vi "Feeding_OPEN_DOOR_ON_SCAN.vi"(7 "CYCLE DATA IN":T1, 8 "error in (no error)":errorcluster, 11 "raw scan code":string) -> (0 "error out":errorcluster, 2 "search valid ?":bool, 5 "CYCLE DATA OUT":T1)   [LabVIEW 2017]
uses:
  Controls/Feed_Cyc_Data.ctl
  <vilib>/Utility/file.llb/Read Delimited Spreadsheet (string).vi
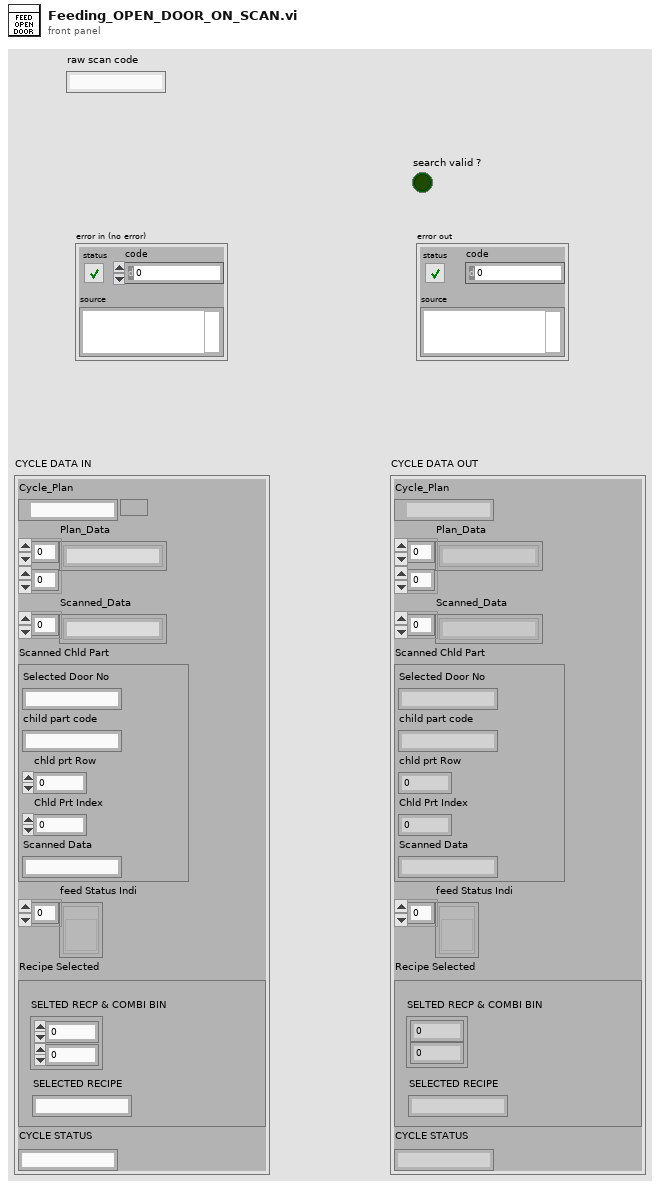
[diagram p1: front panel]
types:
  T1 = typedef "Feed_Cyc_Data.ctl" = cluster{"Cycle_Plan":path, "Plan_Data":string[][], "Scanned_Data":string[], "Scanned Chld Part":cluster{"Selected Door No":string, "child part code":string, "chld prt Row":i32, "Chld Prt Index":i32, "Scanned Data":string}, "feed Status Indi":refnum<vi>[], "Recipe Selected":cluster{"SELTED RECP & COMBI BIN":cluster{i32, i32}, "SELECTED RECIPE":string}, "CYCLE STATUS":string}
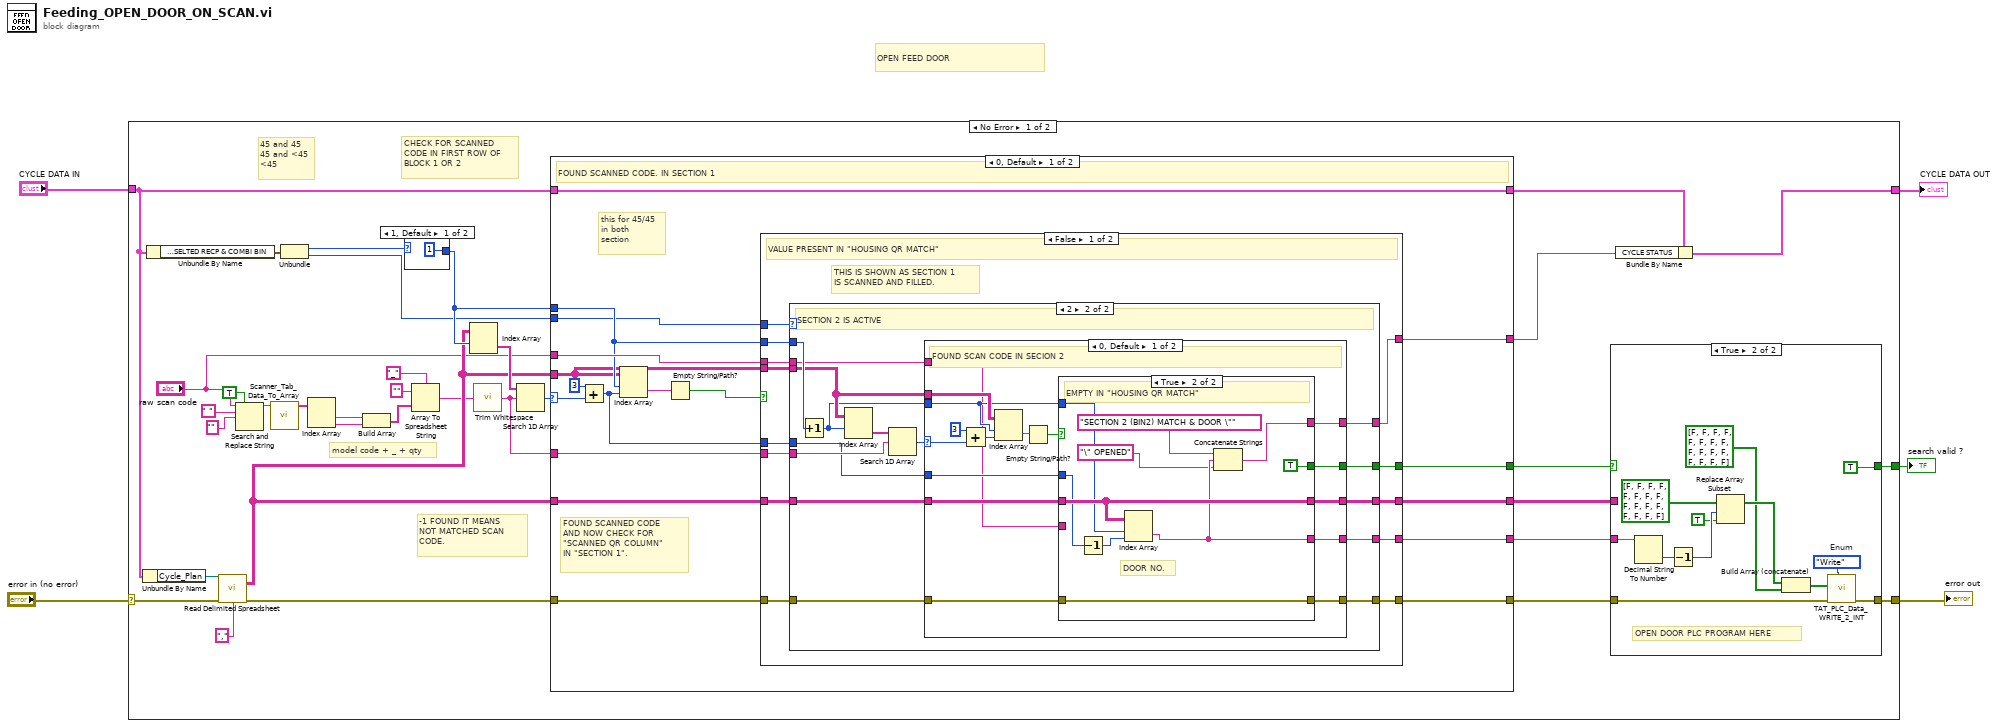
[diagram p0: block diagram]
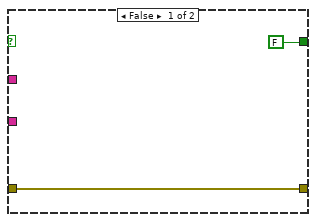
[diagram p2: hidden frame]
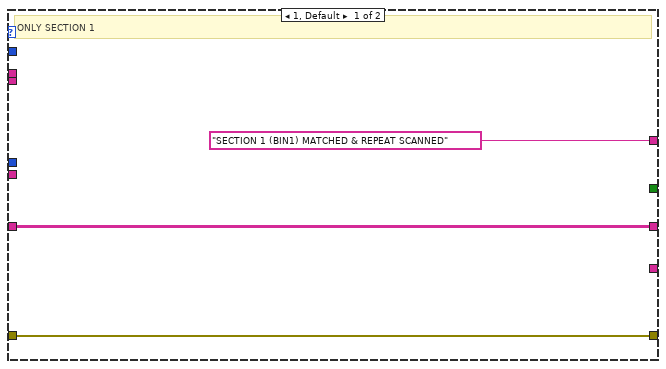
[diagram p3: hidden frame]
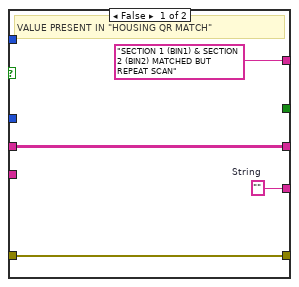
[diagram p4: hidden frame]
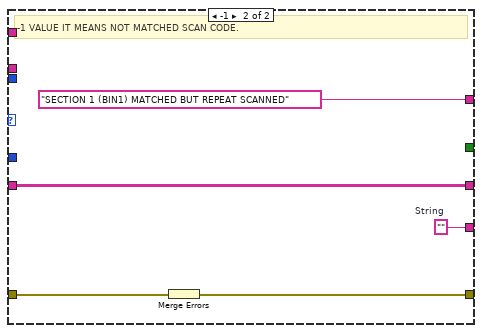
[diagram p5: hidden frame]
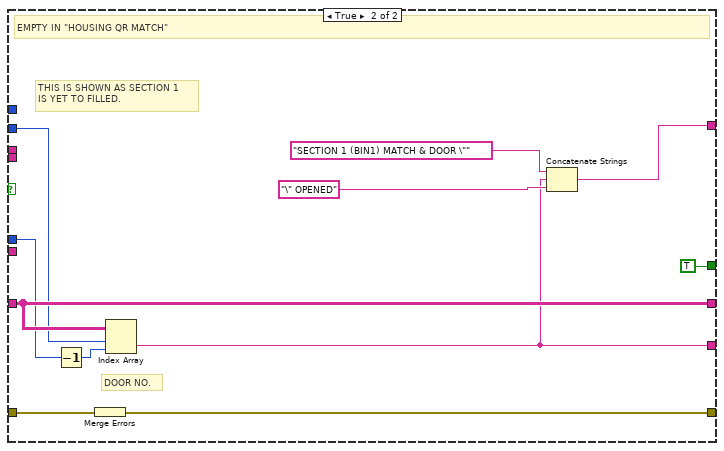
[diagram p6: hidden frame]
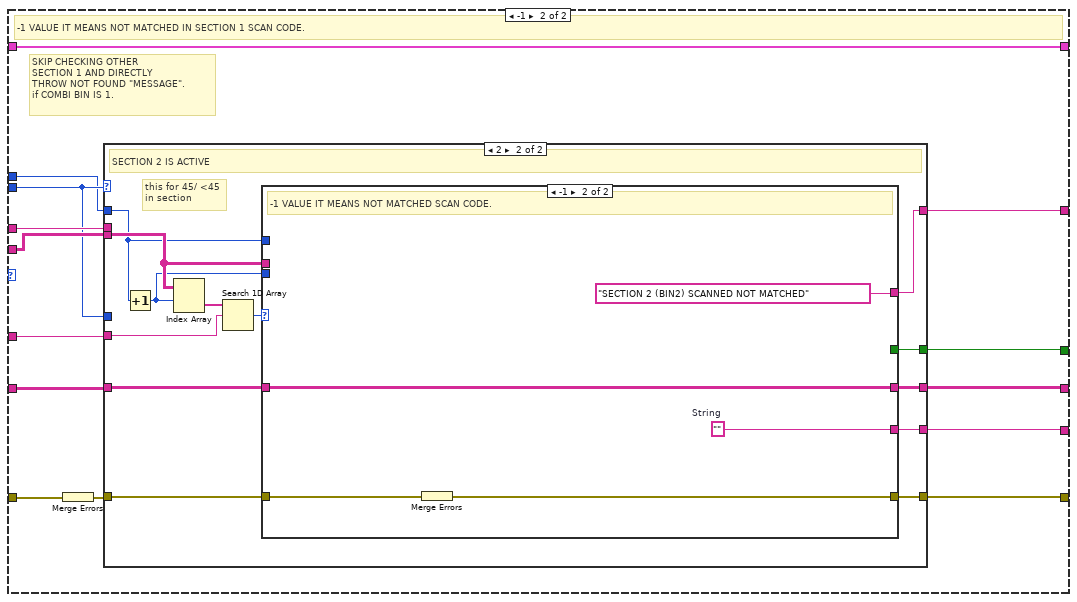
[diagram p7: hidden frame]
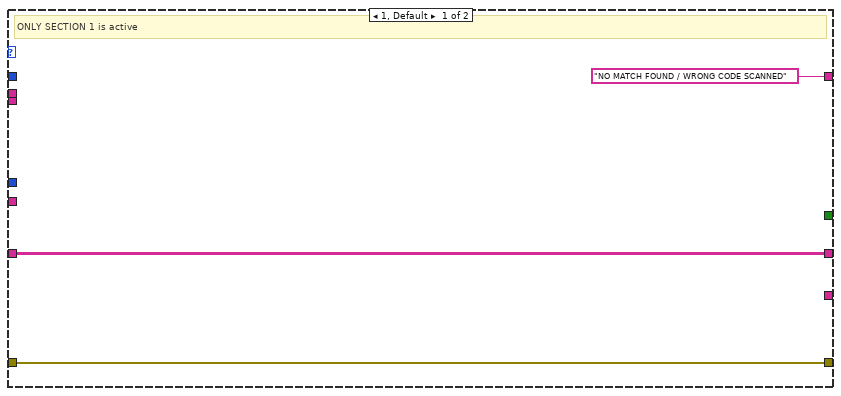
[diagram p8: hidden frame]
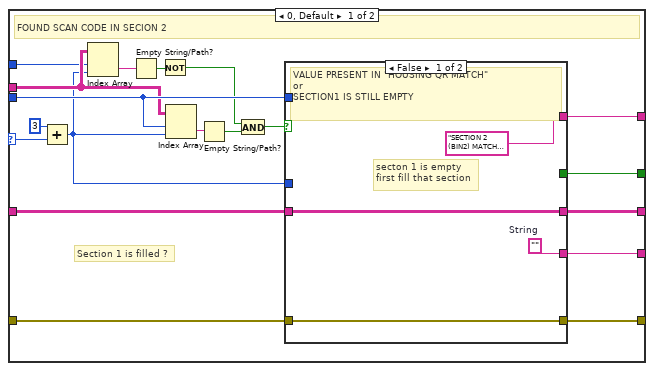
[diagram p9: hidden frame]
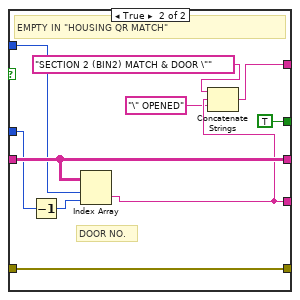
[diagram p10: hidden frame]
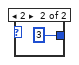
[diagram p11: hidden frame]
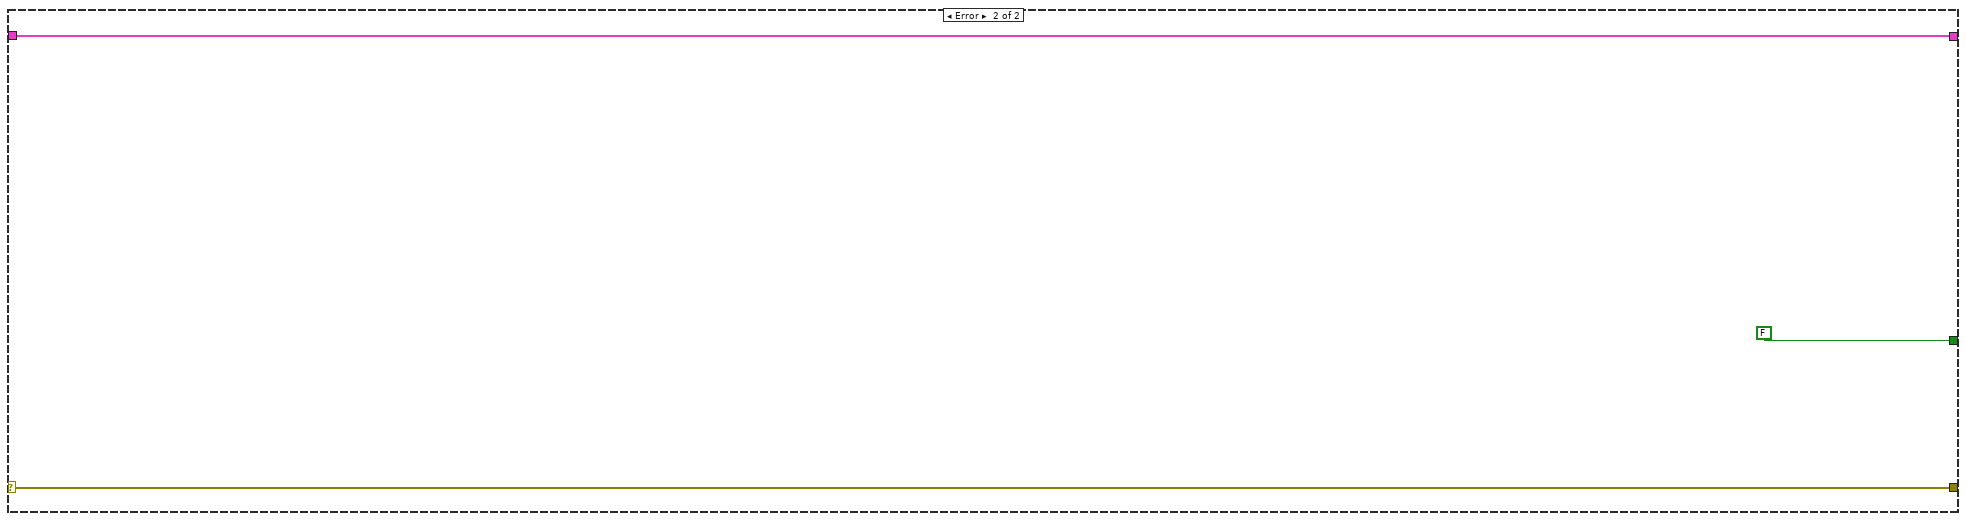
[diagram p12: hidden frame]
diagram:
  # "OPEN FEED DOOR"
  n1 = case shown="No Error" "error in (no error)" {
    selector: "error in (no error)" -> [w36 w221]
    tunnel: [w20 w221] -> w4
    tunnel: [w7 w220] -> w2
    tunnel: "CYCLE DATA IN" -> [w25 w220]
    tunnel: [w11 FALSE] -> w1
    frame No Error {
      # "45 and 45\n45 and <45\n<45"
      # "model code + _ + qty"
      # "-1 FOUND IT MEANS\nNOT MATCHED SCAN\nCODE."
      # "CHECK FOR SCANNED\nCODE IN FIRST ROW OF\nBLOCK 1 OR 2"
      n2 = Unbundle By Name(w25) -> ("Cycle_Plan"=w37:path)
      n3 = Unbundle By Name(w25) -> ("Recipe Selected.SELTED RECP & COMBI BIN"=w34:cluster{i32, i32})
      n4 = call-poly <vilib>:"Read Delimited Spreadsheet.vi"("file path (dialog if empty)"=w37, "error in (no error)"=w36, "delimiter (\\t)"=",") -> ("all rows"=w22:string[][], "error out"=w35:errorcluster)  [unwired: 7 in, 4 out]
      n5 = Search and Replace String(replace all?=TRUE, input string="raw scan code", search string=" ", replace string="") -> (result string=w32:string)  [unwired: 4 in, 3 out]
      n6 = call "Scanner_Tab_Data_To_Array.vi"("Scanner Data"=w32) -> ("Array"=w17:string[])  [unwired: 10 in]
      n7 = Unbundle(w34) -> (w33:i32, w21:i32)
      n8 = Index Array(array=w17) -> (element #1=w16:string, element #2=w15:string)  [unwired: 2 in]
      n9 = Build Array(w16, w15) -> (w14:string[])
      n10 = case shown="1, Default" w33 {
        tunnel: [1 3] -> w23
        frame 1, Default {
        }
        frame 2 {
        }
      }
      n11 = Array To Spreadsheet String(delimiter (Tab)="_", array=w14, 3:"") -> (spreadsheet string=w13:string)
      n12 = Index Array(array=w22, index (row)=w23) -> (element=w26:string[])  [unwired: 1 in]
      n13 = call <vilib>:"Trim Whitespace.vi"("string"=w13) -> ("trimmed string"=w9:string)  [unwired: 1 in]
      n14 = Search 1D Array(1D array=w26, element=w9) -> (index of element=w24:i32)  [unwired: 1 in]
      n15 = case shown="0, Default" w24 {
        selector: w24 -> [w70 _]
        tunnel: [w67 w158] -> w39
        tunnel: w35 -> [w71 w162]
        tunnel: [w64 w161] -> w8
        tunnel: w25 -> [w64 w161]
        tunnel: w22 -> [w58 w153]
        tunnel: w23 -> [w62 w150]
        tunnel: "raw scan code" -> [w65 w154]
        tunnel: w22 -> [w63 w160]
        tunnel: [w60 w156] -> w18
        tunnel: w21 -> [w59 w152]
        tunnel: w9 -> [w57 w151]
        tunnel: [w56 w155] -> w19
        tunnel: [w55 w157] -> w12
        tunnel: [w54 w149] -> w6
        frame 0, Default {
          # "this for 45/45\nin both\nsection"
          # "FOUND SCANNED CODE\nAND NOW CHECK FOR\n\"SCANNED QR COLUMN\"\nIN \"SECTION 1\"."
          # "FOUND SCANNED CODE. IN SECTION 1"
          n16 = Add(x=3, y=w70) -> (x+y=w61:i32)
          n17 = Index Array(array=w58, index (row)=w62, index (col)=w61) -> (element=w68:string)
          n18 = Empty String/Path?(string/path=w68) -> (empty?=w66:bool)
          n19 = case shown="False" w66 {
            tunnel: w71 -> [w83 w148]
            tunnel: [w84 w147] -> w67
            tunnel: w65 -> [w75 _]
            tunnel: w63 -> [w80 w146]
            tunnel: w62 -> [w79 w144]
            tunnel: w61 -> [w77 w143]
            tunnel: [w81 w146] -> w60
            tunnel: w59 -> [w82 _]
            tunnel: w58 -> [w78 _]
            tunnel: w57 -> [w76 _]
            tunnel: [w74 TRUE] -> w56
            tunnel: [w73 w139] -> w55
            tunnel: [w72 w138] -> w54
            frame False {
              # "THIS IS SHOWN AS SECTION 1\nIS SCANNED AND FILLED."
              # "VALUE PRESENT IN \"HOUSING QR MATCH\""
              n20 = case shown="2" w82 {
                tunnel: [w87 w98] -> w84
                tunnel: w83 -> [w87 w102]
                tunnel: [w86 w97] -> w81
                tunnel: w80 -> [w86 w96]
                tunnel: w79 -> [_ w101]
                tunnel: w78 -> [_ w94]
                tunnel: w77 -> [_ w92]
                tunnel: w76 -> [_ w99]
                tunnel: w75 -> [_ w91]
                tunnel: [_ w90] -> w74
                tunnel: [_ w89] -> w73
                tunnel: ["SECTION 1 (BIN1) MATCHED & REPEAT SCANNED" w88] -> w72
                frame 1, Default {
                  # "ONLY SECTION 1"
                }
                frame 2 {
                  # "SECTION 2 IS ACTIVE"
                  n21 = Increment(x=w101) -> (x+1=w93:i32)
                  n22 = Index Array(array=w94, index (row)=w93) -> (element=w100:string[])  [unwired: 1 in]
                  n23 = Search 1D Array(1D array=w100, element=w99) -> (index of element=w95:i32)  [unwired: 1 in]
                  n24 = case shown="0, Default" w95 {
                    selector: w95 -> [w115 _]
                    tunnel: w102 -> [w118 w137]
                    tunnel: [w113 w136] -> w98
                    tunnel: [w110 w135] -> w97
                    tunnel: w96 -> [w109 w135]
                    tunnel: w94 -> [w114 _]
                    tunnel: w93 -> [w108 _]
                    tunnel: w92 -> [w107 _]
                    tunnel: w91 -> [w106 _]
                    tunnel: [w105 _] -> w90
                    tunnel: [w104 w134] -> w89
                    tunnel: [w103 "SECTION 1 (BIN1) MATCHED BUT REPEAT SCANNED"] -> w88
                    frame 0, Default {
                      # "FOUND SCAN CODE IN SECION 2"
                      n25 = Add(x=3, y=w115) -> (x+y=w117:i32)
                      n26 = Index Array(array=w114, index (row)=w108, index (col)=w117) -> (element=w112:string)
                      n27 = Empty String/Path?(string/path=w112) -> (empty?=w111:bool)
                      n28 = case shown="True" w111 {
                        tunnel: w118 -> [w121 w132]
                        tunnel: [w121 w132] -> w113
                        tunnel: [w122 w129] -> w110
                        tunnel: w109 -> [w122 w129]
                        tunnel: w108 -> [_ w128]
                        tunnel: w107 -> [_ w127]
                        tunnel: w106 -> [_ _]
                        tunnel: [_ TRUE] -> w105
                        tunnel: [w120 w125] -> w104
                        tunnel: ["SECTION 1 (BIN1) & SECTION 2 (BIN2) MATCHED BUT REPEAT SCAN" w123] -> w103
                        frame False {
                          w120 = ""  # String
                          # "VALUE PRESENT IN \"HOUSING QR MATCH\""
                        }
                        frame True {
                          # "DOOR NO."
                          # "EMPTY IN \"HOUSING QR MATCH\""
                          n29 = Decrement(x=w127) -> (x-1=w130:i32)
                          n30 = Index Array(array=w129, index (row)=w128, index (col)=w130) -> (element=w125:string)
                          n31 = Concatenate Strings("SECTION 2 (BIN2) MATCH & DOOR \"", w125, "\" OPENED") -> (w123:string)
                        }
                      }
                    }
                    frame -1 {
                      w134 = ""  # String
                      # "-1 VALUE IT MEANS NOT MATCHED SCAN CODE."
                      n32 = Merge Errors(w137) -> (w136:errorcluster)
                    }
                  }
                }
              }
            }
            frame True {
              # "DOOR NO."
              # "THIS IS SHOWN AS SECTION 1\nIS YET TO FILLED."
              # "EMPTY IN \"HOUSING QR MATCH\""
              n33 = Decrement(x=w143) -> (x-1=w142:i32)
              n34 = Merge Errors(w148) -> (w147:errorcluster)
              n35 = Index Array(array=w146, index (row)=w144, index (col)=w142) -> (element=w139:string)
              n36 = Concatenate Strings("SECTION 1 (BIN1) MATCH & DOOR \"", w139, "\" OPENED") -> (w138:string)
            }
          }
        }
        frame -1 {
          # "SKIP CHECKING OTHER \nSECTION 1 AND DIRECTLY\nTHROW NOT FOUND \"MESSAGE\". \nif COMBI BIN IS 1."
          # "-1 VALUE IT MEANS NOT MATCHED IN SECTION 1 SCAN CODE."
          n37 = Merge Errors(w162) -> (w159:errorcluster)
          n38 = case shown="2" w152 {
            tunnel: [w165 w176] -> w158
            tunnel: w159 -> [w165 w178]
            tunnel: [w164 w175] -> w156
            tunnel: w160 -> [w164 w174]
            tunnel: w153 -> [_ w171]
            tunnel: w152 -> [_ _]
            tunnel: w151 -> [_ w177]
            tunnel: w154 -> [_ _]
            tunnel: [_ w173] -> w155
            tunnel: [_ w172] -> w157
            tunnel: w150 -> [_ w167]
            tunnel: ["NO MATCH FOUND / WRONG CODE SCANNED" w166] -> w149
            frame 1, Default {
              # "ONLY SECTION 1 is active"
            }
            frame 2 {
              # "this for 45/ <45\nin section"
              # "SECTION 2 IS ACTIVE"
              n39 = Increment(x=w167) -> (x+1=w168:i32)
              n40 = Index Array(array=w171, index (row)=w168) -> (element=w170:string[])  [unwired: 1 in]
              n41 = Search 1D Array(1D array=w170, element=w177) -> (index of element=w169:i32)  [unwired: 1 in]
              n42 = case shown="-1" w169 {
                selector: w169 -> [w195 _]
                tunnel: w178 -> [w197 w216]
                tunnel: [w194 w215] -> w176
                tunnel: [w191 w214] -> w175
                tunnel: w174 -> [w190 w214]
                tunnel: w171 -> [w186 _]
                tunnel: w168 -> [w189 _]
                tunnel: [w188 _] -> w173
                tunnel: [w187 w213] -> w172
                tunnel: w167 -> [w185 _]
                tunnel: [w179 "SECTION 2 (BIN2) SCANNED NOT MATCHED"] -> w166
                frame 0, Default {
                  # "Section 1 is filled ?"
                  # "FOUND SCAN CODE IN SECION 2"
                  n43 = Add(x=3, y=w195) -> (x+y=w184:i32)
                  n44 = Index Array(array=w186, index (row)=w185, index (col)=w184) -> (element=w183:string)
                  n45 = Empty String/Path?(string/path=w183) -> (empty?=w182:bool)
                  n46 = Not(x=w182) -> (.not. x?=w180:bool)
                  n47 = Index Array(array=w186, index (row)=w189, index (col)=w184) -> (element=w193:string)
                  n48 = Empty String/Path?(string/path=w193) -> (empty?=w192:bool)
                  n49 = And(x=w180, y=w192) -> (x .and. y?=w181:bool)
                  n50 = case shown="False" w181 {
                    tunnel: w197 -> [w200 w211]
                    tunnel: [w200 w211] -> w194
                    tunnel: [w201 w208] -> w191
                    tunnel: w190 -> [w201 w208]
                    tunnel: w189 -> [_ w207]
                    tunnel: w184 -> [_ w206]
                    tunnel: [_ TRUE] -> w188
                    tunnel: [w199 w204] -> w187
                    tunnel: ["SECTION 2 (BIN2) MATCH BUT - SECTION 1 NOT SCANED YET OR SECTION REPEAT SCANNED" w202] -> w179
                    frame False {
                      w199 = ""  # String
                      # "secton 1 is empty\nfirst fill that section"
                      # "VALUE PRESENT IN \"HOUSING QR MATCH\"\nor\nSECTION1 IS STILL EMPTY"
                    }
                    frame True {
                      # "DOOR NO."
                      # "EMPTY IN \"HOUSING QR MATCH\""
                      n51 = Decrement(x=w206) -> (x-1=w209:i32)
                      n52 = Index Array(array=w208, index (row)=w207, index (col)=w209) -> (element=w204:string)
                      n53 = Concatenate Strings("SECTION 2 (BIN2) MATCH & DOOR \"", w204, "\" OPENED") -> (w202:string)
                    }
                  }
                }
                frame -1 {
                  w213 = ""  # String
                  # "-1 VALUE IT MEANS NOT MATCHED SCAN CODE."
                  n54 = Merge Errors(w216) -> (w215:errorcluster)
                }
              }
            }
          }
        }
      }
      n55 = case shown="True" w19 {
        tunnel: w39 -> [w41 w47]
        tunnel: [w41 w46] -> w20
        tunnel: w18 -> [_ _]
        tunnel: w12 -> [_ w53]
        tunnel: [FALSE TRUE] -> w11
        frame False {
        }
        frame True {
          w52 = enum16{"Read", "Write"}."Write"  # Enum
          # "OPEN DOOR PLC PROGRAM HERE"
          n56 = Decimal String To Number(string=w53) -> (number=w48:i32)  [unwired: 2 in, 1 out]
          n57 = Decrement(x=w48) -> (x-1=w50:i32)
          n58 = Replace Array Subset(array=bool[] [FALSE, FALSE, FALSE, FALSE, FALSE, FALSE, FALSE, FALSE, FALSE, FALSE, FALSE, FALSE, FALSE, FALSE, FALSE, FALSE], new element=TRUE, index=w50) -> (w44:bool[])
          n59 = Build Array (concatenate)(w44, bool[] [FALSE, FALSE, FALSE, FALSE, FALSE, FALSE, FALSE, FALSE, FALSE, FALSE, FALSE, FALSE, FALSE, FALSE, FALSE, FALSE]) -> (w45:bool[])
          n60 = call "TAT_PLC_Data_WRITE_2_INT.vi"("Enum"=w52, "error in (no error)"=w47, "Array"=w45) -> ("error out"=w46:errorcluster)  [unwired: 7 in, 1 out]
        }
      }
      n61 = Bundle By Name(cluster=w8, "CYCLE STATUS"=w6) -> (w7:T1)
    }
    frame Error {
    }
  }
  "error out" <- w4
  "CYCLE DATA OUT" <- w2
  "search valid ?" <- w1
